vi "Config Seq & Error.vi"(8 "error in (no error)":errorcluster, 11 "Sequences":T1) -> (0 "error out":errorcluster, 3 "Sequences":T1)   [LabVIEW 2014, in "SeqLoop.lvlib"]
uses:
  SeqLoop.lvlib
  TypeDefs/Sequence.ctl
  Classes/STEP/STEP.lvclass
  TypeDefs/LogicParsedExpression.ctl
panel:
  in  "Save":bool
  in  "Close":bool
  in  "Config AutoZero":bool
  in  "Error&Alarms":bool
  # "Elija la opción que desea configurar"
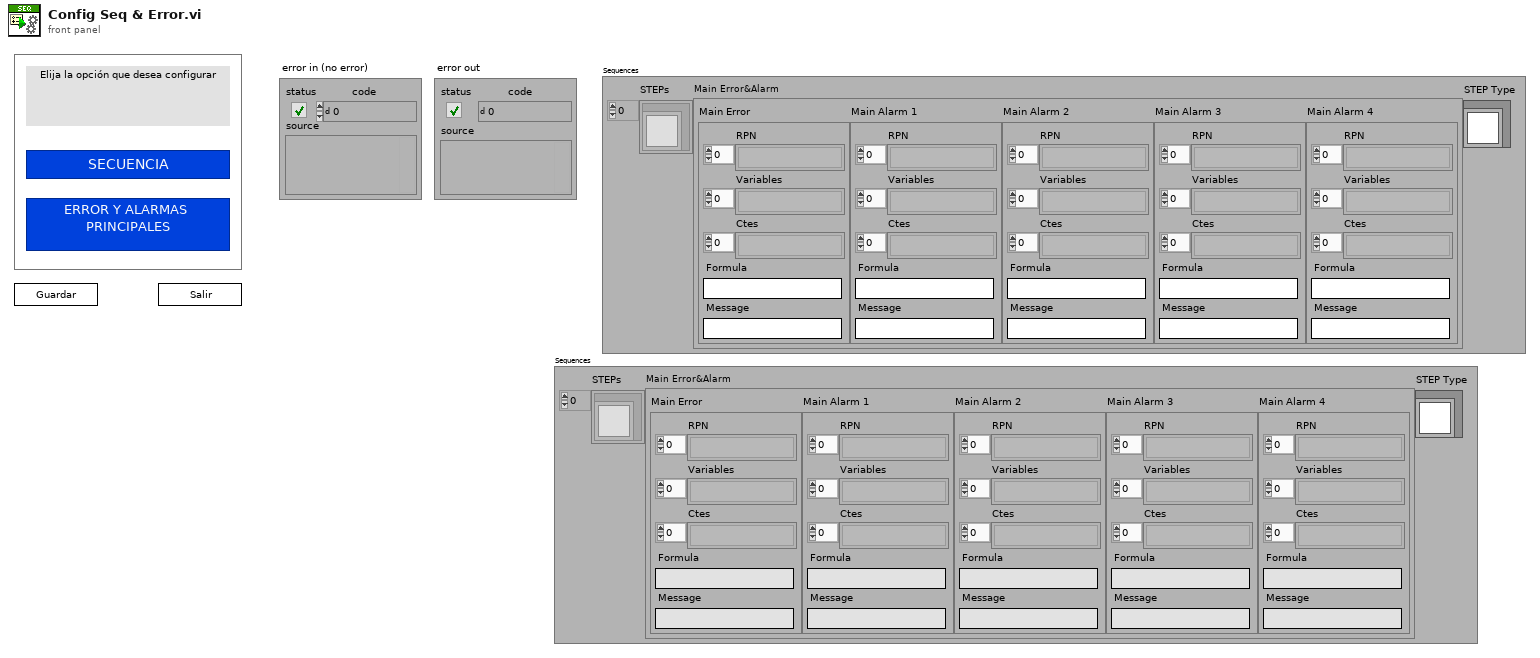
[diagram p1: front panel]
types:
  T1 = typedef "SeqLoop.lvlib/Sequence.ctl" = cluster{"STEPs":refnum<class "STEP.lvclass">[], "Main Error&Alarm":cluster{"Main Error":T2, "Main Alarm 1":T2, "Main Alarm 2":T2, "Main Alarm 3":T2, "Main Alarm 4":T2}, "STEP Type":refnum<class "STEP.lvclass">}
  T2 = typedef "SeqLoop.lvlib/LogicParsedExpression.ctl" = cluster{"RPN ":string[], "Variables":string[], "Ctes":string[], "Formula":string, "Message":string}
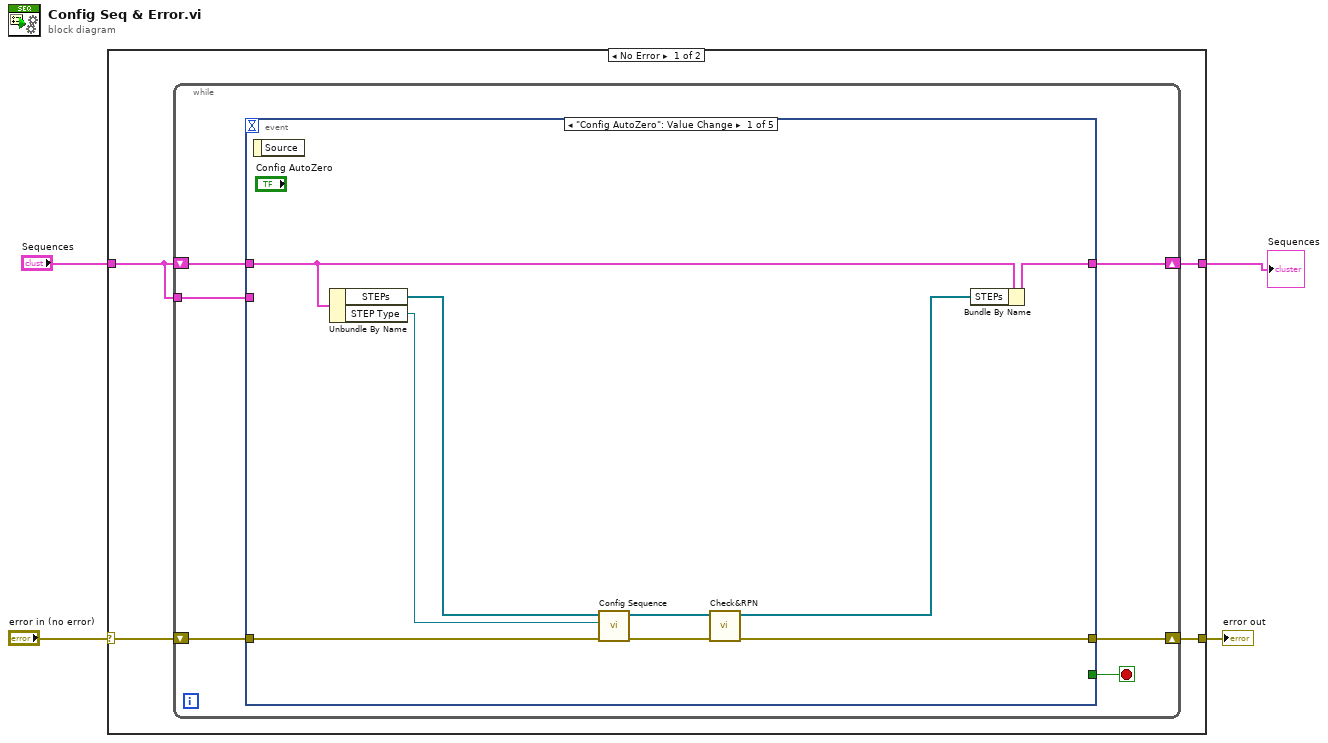
[diagram p0: block diagram]
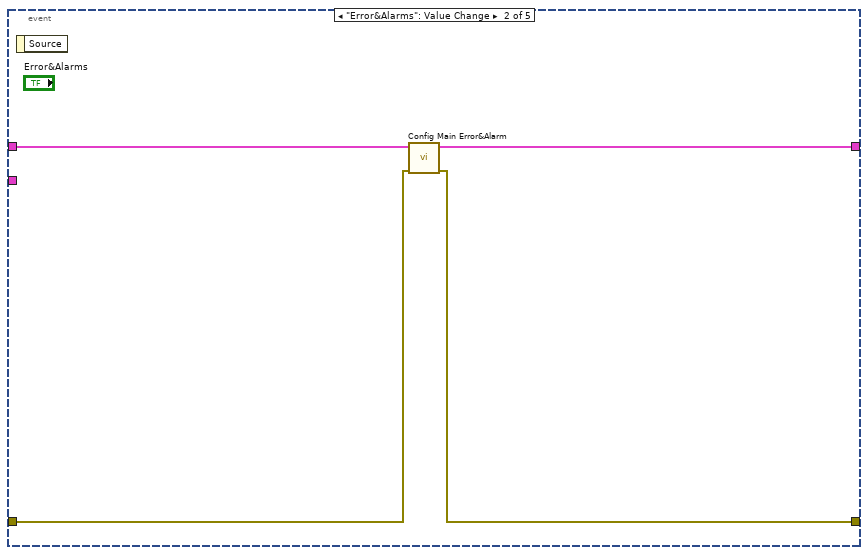
[diagram p2: hidden frame]
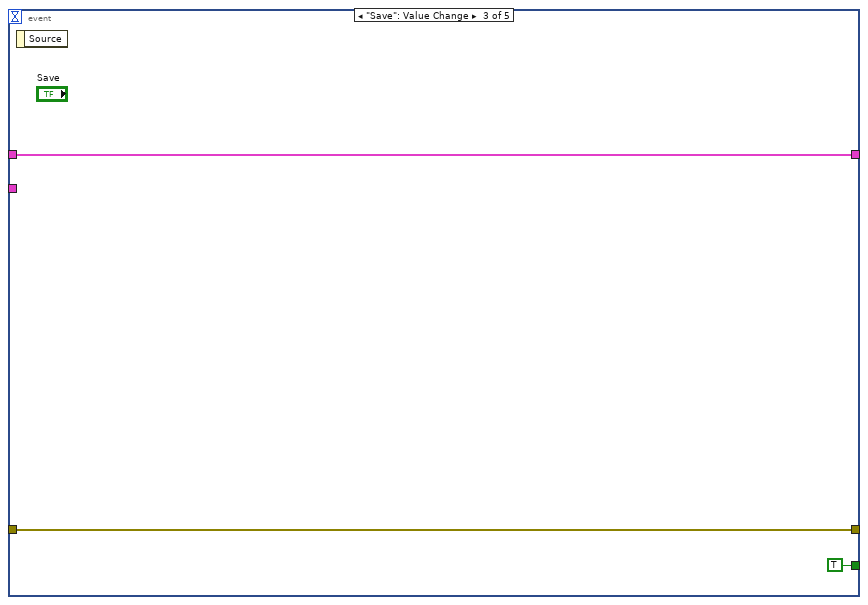
[diagram p3: hidden frame]
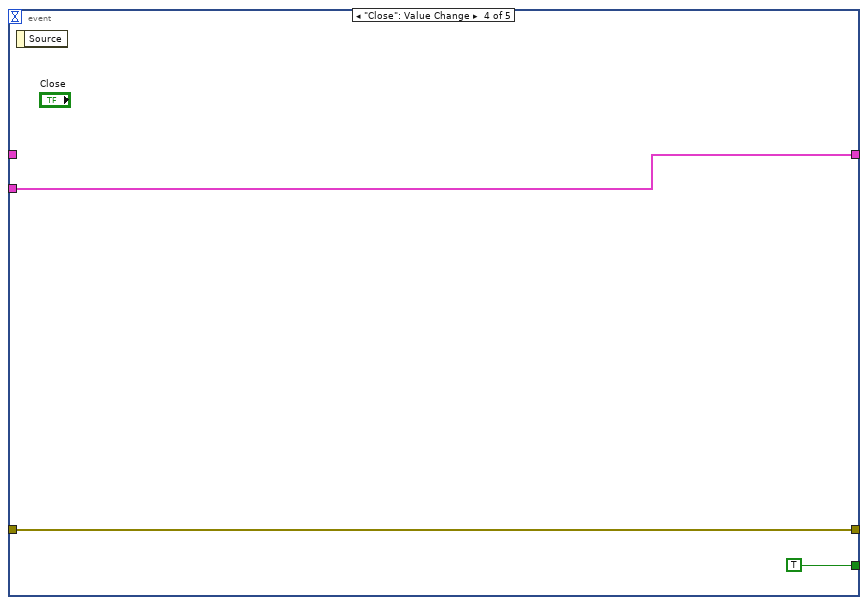
[diagram p4: hidden frame]
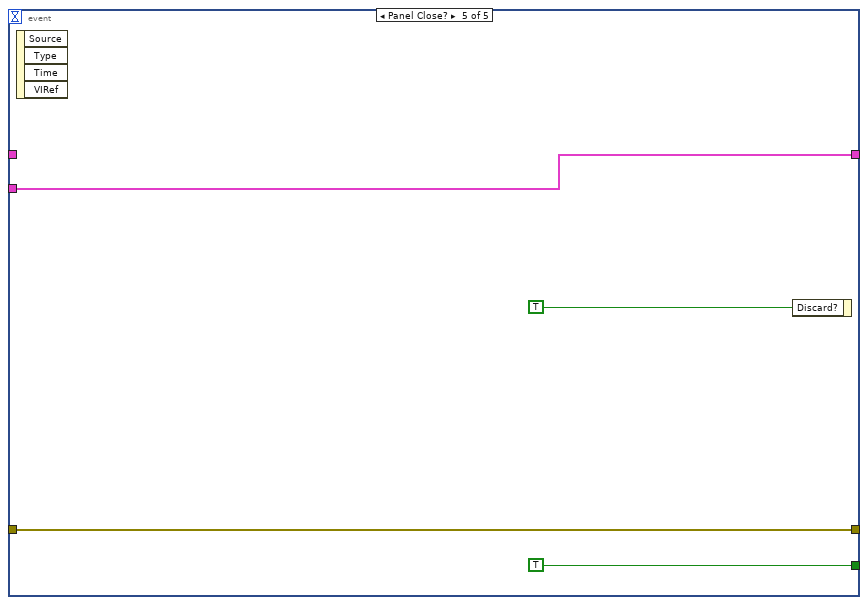
[diagram p5: hidden frame]
diagram:
  n1 = case shown="No Error" "error in (no error)" {
    selector: "error in (no error)" -> [w8 w39]
    tunnel: [w7 w39] -> w3
    tunnel: [w6 w38] -> w2
    tunnel: "Sequences" -> [w5 w38]
    frame No Error {
      n2 = while {
        shift-right: [w13] -> w7
        shift-left: w8 -> [w14]
        shift-right: [w12] -> w6
        shift-left: w5 -> [w11]
        tunnel: w5 -> [w9]
        stop <- w10 stop-if-true
        n3 = event shown="[0] \"Config AutoZero\": Value Change" {
          selector: _ -> [_ _ _ _ _]
          dyn-events: _ -> [_ _ _ _ _]
          timeout: _ -> [_ _ _ _ _]
          tunnel: w14 -> [w22 w24 w28 w33 w35]
          tunnel: [w21 w25 w28 w33 w35] -> w13
          tunnel: [w20 w26 w30 w31 w34] -> w12
          tunnel: w11 -> [w19 w27 w30 _ _]
          tunnel: [_ _ TRUE TRUE TRUE] -> w10
          tunnel: w9 -> [_ _ _ w31 w34]
          event "Config AutoZero": Value Change {
            n4 = event-data() -> ()  [unwired: 1 in, 1 out]
            n5 = Unbundle By Name(w19) -> ("STEPs"=w18:refnum<class "STEP.lvclass">[], "STEP Type"=w15:refnum<class "STEP.lvclass">)
            n6 = call "Config Sequence.vi"("error in (no error)"=w22, "new element/subarray"=w15, "All Sequence STEPs in"=w18) -> ("error out"=w23:errorcluster, "All Sequence STEPs"=w17:refnum<class "STEP.lvclass">[])  [unwired: 7 in]
            n7 = call "Check&RPN.vi"("error in (no error)"=w23, "Array STEP"=w17) -> ("error out"=w21:errorcluster, "STEP Out"=w16:refnum<class "STEP.lvclass">[])  [unwired: 8 in]
            n8 = Bundle By Name(cluster=w19, "STEPs"=w16) -> (w20:T1)
          }
          event "Error&Alarms": Value Change {
            n9 = event-data() -> ()  [unwired: 1 in, 1 out]
            n10 = call "Config Main Error&Alarm.vi"("error in (no error)"=w24, "Sequence"=w27) -> ("error out"=w25:errorcluster, "Sequence out"=w26:T1)  [unwired: 8 in]
          }
          event "Save": Value Change {
            n11 = event-data() -> ()  [unwired: 1 in, 1 out]
          }
          event "Close": Value Change {
            n12 = event-data() -> ()  [unwired: 1 in, 1 out]
          }
          event Panel Close? {
            n13 = event-data() -> ()  [unwired: 1 in, 4 out]
            n14 = event-data("Discard?"=TRUE) -> ()  [unwired: 1 in, 1 out]
          }
        }
      }
    }
    frame Error {
    }
  }
  "error out" <- w3
  "Sequences" <- w2
